vi "Write 7z.bat.vi"(8 "error in (no error)":errorcluster, 11 "PostBuildSupport in":refnum<class "PostBuildSupport (2013).lvclass">) -> (0 "error out":errorcluster, 3 "PostBuildSupport out":refnum<class "PostBuildSupport (2013).lvclass">)   [LabVIEW 2016, in "PostBuildSupport (2013).lvclass"]
uses:
  PostBuildSupport (2013).lvclass
  PostBuildSupport (2013).lvclass/PostBuildSupport (2013).ctl
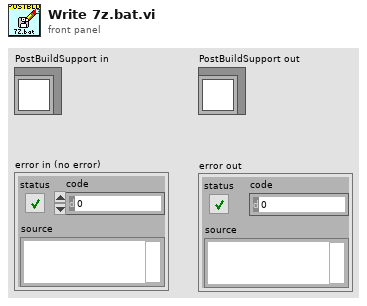
[diagram p1: front panel]
types:
  T1 = enum16{"open", "replace", "create", "open or create", "replace or create", "replace or create with confirmation"}
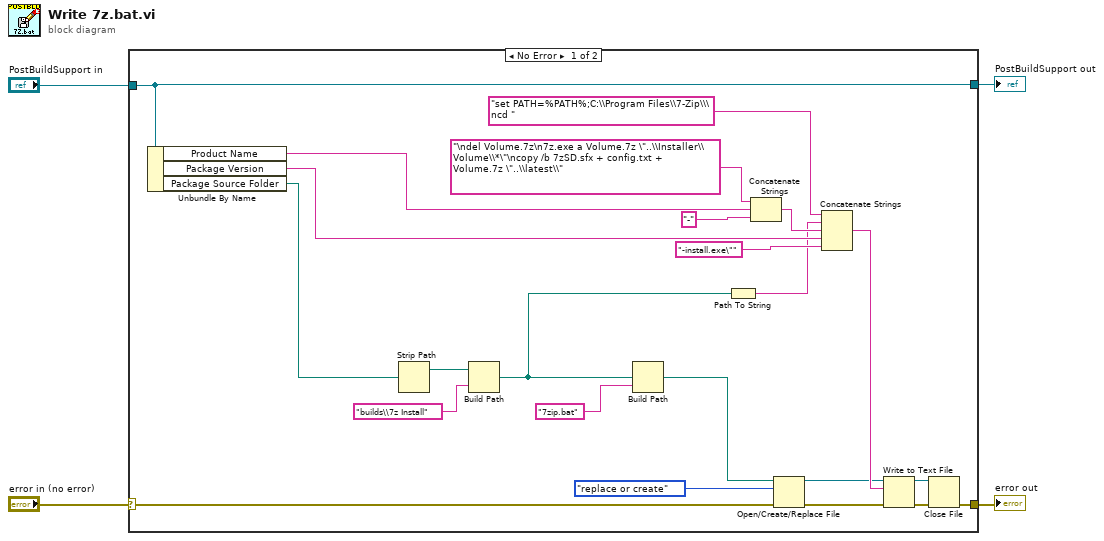
[diagram p0: block diagram]
diagram:
  n1 = case shown="No Error" "error in (no error)" {
    selector: "error in (no error)" -> [w8 w29]
    tunnel: [w17 w29] -> w4
    tunnel: "PostBuildSupport in" -> [w7 w28]
    tunnel: [w7 w28] -> w1
    frame No Error {
      n2 = Unbundle By Name(w7) -> ("Product Name"=w9:string, "Package Version"=w12:string, "Package Source Folder"=w11:path)
      n3 = Strip Path(path=w11) -> (stripped path=w24:path)  [unwired: 1 out]
      n4 = Build Path(base path=w24, name or relative path="builds\\7z Install") -> (appended path=w6:path)
      n5 = Build Path(base path=w6, name or relative path="7zip.bat") -> (appended path=w22:path)
      n6 = Path To String(path=w6) -> (string=w5:string)
      n7 = Concatenate Strings("\ndel Volume.7z\n7z.exe a Volume.7z \"..\\Installer\\Volume\\*\"\ncopy /b 7zSD.sfx + config.txt + Volume.7z \"..\\latest\\" ("Name of target (My Computer)"), w9, "-" ("Name of target (My Computer)")) -> (w14:string)
      n8 = Open/Create/Replace File(file path (use dialog)=w22, error in=w8, operation (0:open)=T1."replace or create") -> (refnum out=w23:refnum<file>, error out=w21:errorcluster)  [unwired: 3 in, 1 out]
      n9 = Concatenate Strings("set PATH=%PATH%;C:\\Program Files\\7-Zip\\\ncd " ("Name of target (My Computer)"), w5, w14, w12, "-install.exe\"" ("Name of target (My Computer)")) -> (w27:string)
      n10 = Write to Text File(file (use dialog)=w23, text=w27, error in=w21) -> (refnum out=w18:refnum<file>, error out=w19:errorcluster)  [unwired: 1 in, 1 out]
      n11 = Close File(refnum=w18, error in=w19) -> (error out=w17:errorcluster)  [unwired: 1 out]
    }
    frame Error {
    }
  }
  "error out" <- w4
  "PostBuildSupport out" <- w1
